vi "sub_rad_to_deg.vi"(11 "rad in":dbl) -> (3 "deg out":dbl)   [LabVIEW 2019]
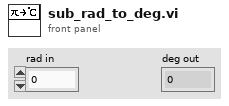
[diagram p1: front panel]
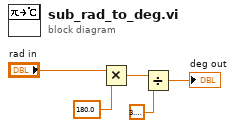
[diagram p0: block diagram]
diagram:
  n1 = Multiply(x="rad in", y=180.0) -> (x*y=w3:dbl)
  n2 = Divide(x=w3, y=3.141592653589793) -> (x/y=→"deg out":dbl)
